vi "fft_demodulator.vi"(0 "Reset":bool, 5 "Config":T2={"IO params"={"Conversion"={"Rate"=4.0, "Num cards"=2, "Out channels"=4}, "Carriers"={"Phase shift"=180.0, "Levels"=[[0.8, 0.8, 0.8], [0.03, 0.03, 0.03]], "Delay samples"=73.15}, "TCP"={"Host"="192.168.1.15", "Port"=6666, "Buffering"=6, "Timeout"=6}, "Input channel sign"=[1, 1, 1]}, "High rate STFT"={"Win param"=101.5, "Window type"=61, "Win order"=2, "DFT size"=64, "Channels"=[7], "Oversample"=64}, "Low rate STFT"={"Win param"=120.0, "Window type"=61, "Win order"=8, "DFT size"=64, "Channels"=[7], "Oversample"=64}, "Filtering "=[]} {"Filtering"."Distortion"."Limit" format="%#_3p"; "Filtering"."Distortion"."LF cut" format="%#_3p"; "Filtering"."Kalman"."Measure noise" format="%#_3p"; "Filtering"."Kalman"."Process noise" format="%#_3p"; "Filtering"."Hum"."Limit" format="%#_3p"; "Filtering"."Hum"."Frequency" format="%#_4p"; "Low rate STFT"."Oversample" min=1 step=1; "Low rate STFT"."Channels" min=0 step=1; "Low rate STFT"."DFT size" min=1 step=1; "Low rate STFT"."Window type" items=["Rectangle"=0, "Hanning"=1, "Hamming"=2, "Blackman-Harris"=3, "Exact Blackman"=4, "Blackman"=5, "Flat Top"=6, "4 Term B-Harris "=7, "7 Term B-Harris"=8, "Low Sidelobe"=9, "Blackman Nuttall"=11, "Triangle"=30, "Bartlett-Hanning"=31, "Bohman"=32, "Parzen"=33, "Welch"=34, "Kaiser"=60, "Dolph-Chebyshev"=61, "Gaussian"=62]; "High rate STFT"."Oversample" min=1 step=1; "High rate STFT"."Channels" min=0 step=1; "High rate STFT"."DFT size" min=1 step=1; "High rate STFT"."Window type" items=["Rectangle"=0, "Hanning"=1, "Hamming"=2, "Blackman-Harris"=3, "Exact Blackman"=4, "Blackman"=5, "Flat Top"=6, "4 Term B-Harris "=7, "7 Term B-Harris"=8, "Low Sidelobe"=9, "Blackman Nuttall"=11, "Triangle"=30, "Bartlett-Hanning"=31, "Bohman"=32, "Parzen"=33, "Welch"=34, "Kaiser"=60, "Dolph-Chebyshev"=61, "Gaussian"=62]; "IO params"."Input channel sign" min=-1 max=1 step=1; "IO params"."Carriers"."Levels" min=0.0 step=0.1; "IO params"."Conversion"."Rate" format="%#_8g"}, 7 "Modulation info":T8={"Fs full"=0.0, "Fs high"=0.0, "Fs low"=0.0, "Read size"=0, "FFT size low"=5000, "df low"=5000.0, "High carriers"=[], "Low carriers"=[], "Hi channels at low"=[7]} {"Hi channels at low" min=0 step=1; "Low carriers" format="%#_6p"; "High carriers" format="%#_6p"}, 9 "Low carrier amplitudes":cdb[](array[numeric]) format="%#_3p", 12 "Raw data":dbl[](array[numeric]), 13 "Current/sensor index":i32 min=0 max=1 step=1) -> (10 "High carrier amplitudes":cdb[][](array[numeric]) format="%_3p", 15 "Trace channel out":T1)   [LabVIEW 2026]
uses:
  modulation_info.ctl
  ilemt_config.ctl
  system/IO_params.ctl
  stft_params.ctl
  <vilib>/Analysis/4window.llb/windowTd.ctl
  filter_params.ctl
  detrend_mode.ctl
  gui/trace_channel.ctl
  <vilib>/Analysis/NI_AALPro.lvlib
panel:
  out "DIstortion filter attenuation":dbl
  out "Distortion filter RMS":dbl[](array[numeric])
  out "Distortion filter":dbl[][](graph)
  # "This VI deals with high-rate demodulation and filtering for a single sensor axis."
  # "Rows are time (high carrier samples), columns are high rate source XYZ axis amplitudes."
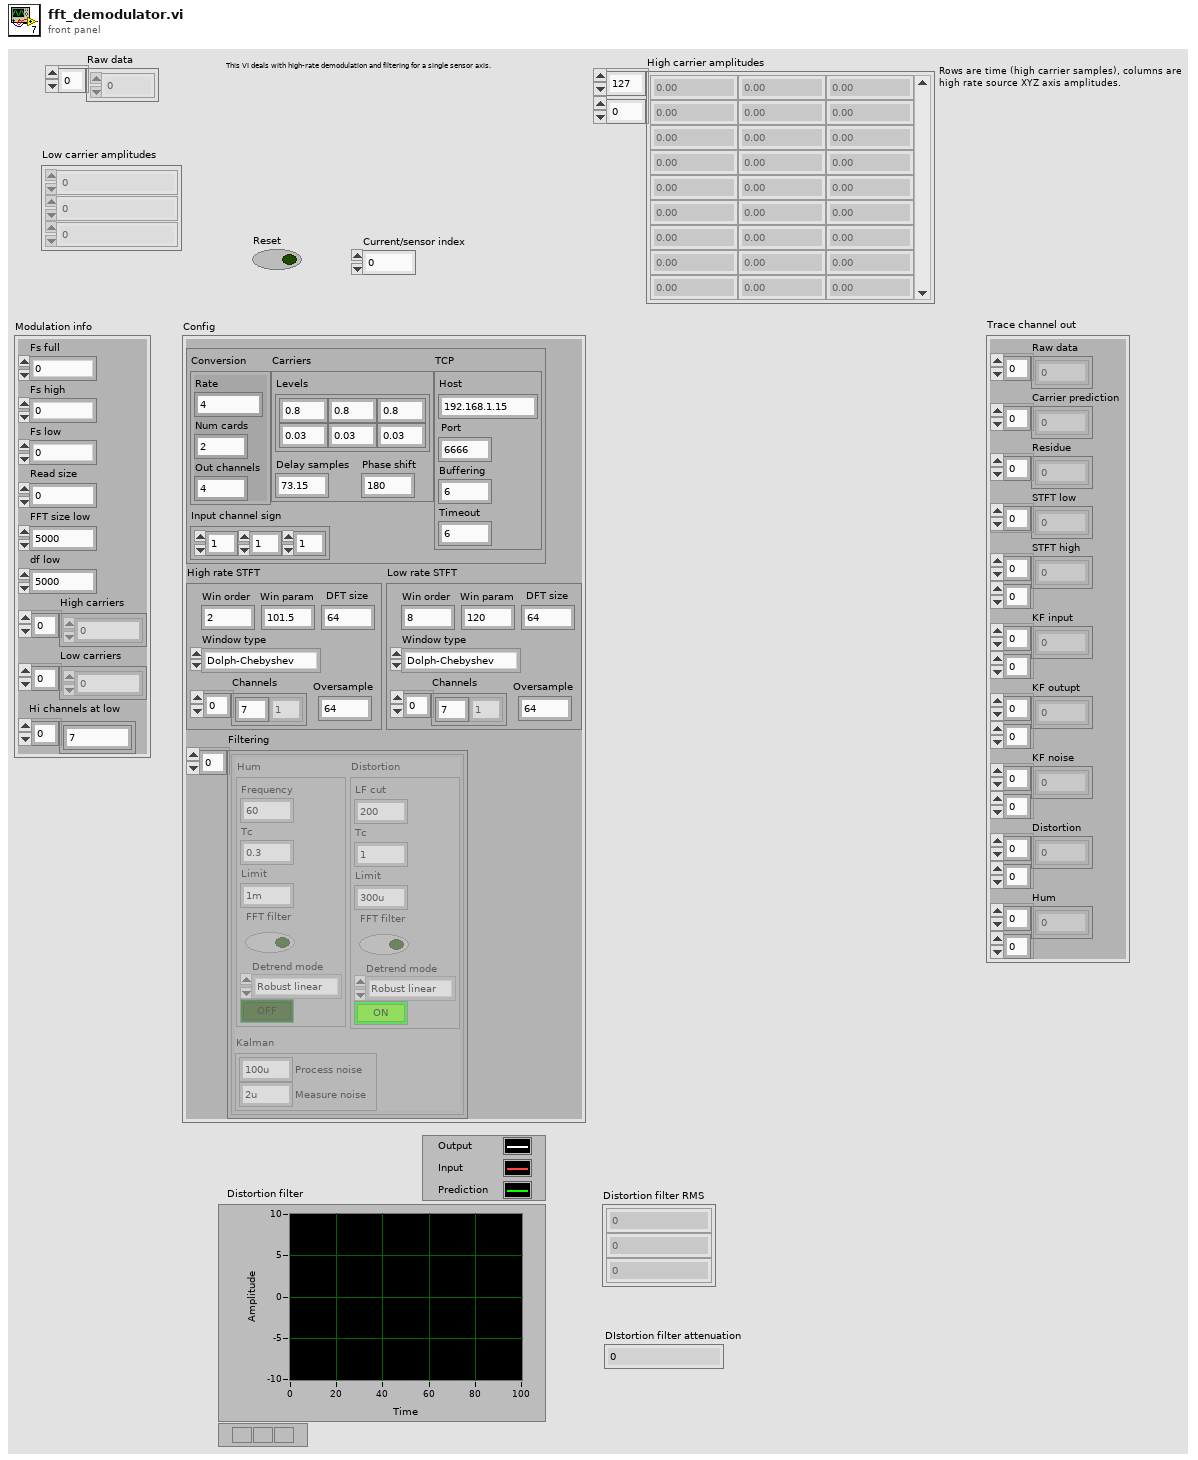
[diagram p1: front panel]
types:
  T1 = typedef "trace_channel.ctl" = cluster{"Raw data":dbl[], "Carrier prediction":dbl[], "Residue":dbl[], "STFT low":cdb[], "STFT high":cdb[][], "KF input":cdb[][], "KF outupt":cdb[][], "KF noise":dbl[][], "Distortion":cdb[][], "Hum":cdb[][]}
  T2 = typedef "ilemt_config.ctl" = cluster{"IO params":T3, "High rate STFT":T4, "Low rate STFT":T4, "Filtering ":T6[]}
  T3 = typedef "IO_params.ctl" = cluster{"Conversion":cluster{"Rate":dbl, "Num cards":u32, "Out channels":u32}, "Carriers":cluster{"Phase shift":dbl, "Levels":dbl[][], "Delay samples":dbl}, "TCP":cluster{"Host":string, "Port":i32, "Buffering":u32, "Timeout":u32}, "Input channel sign":i32[]}
  T4 = typedef "stft_params.ctl" = cluster{"Win param":dbl, "Window type":T5, "Win order":i32, "DFT size":i32, "Channels":i32[], "Oversample":i32}
  T5 = typedef "NI_AALPro.lvlib/windowTd.ctl" = u32
  T6 = typedef "filter_params.ctl" = cluster{"Hum":cluster{"Frequency":dbl, "Tc":dbl, "Limit":dbl, "FFT filter":bool, "Detrend mode":T7, "Enable":bool}, "Kalman":cluster{"Process noise":dbl, "Measure noise":dbl}, "Distortion":cluster{"LF cut":dbl, "Tc":dbl, "Limit":dbl, "FFT filter":bool, "Detrend mode":T7, "Enable":bool}}
  T7 = typedef "detrend_mode.ctl" = enum16{"Zero mean", "Linear", "Robust linear"}
  T8 = typedef "modulation_info.ctl" = cluster{"Fs full":dbl, "Fs high":dbl, "Fs low":dbl, "Read size":i32, "FFT size low":i32, "df low":dbl, "High carriers":dbl[], "Low carriers":dbl[], "Hi channels at low":i32[]}
  T9 = typedef "averaging_filter_params.ctl" = cluster{"Order":i32, "Time constant":dbl, "Detrend mode":T7, "TD amplitude limit":dbl, "FFT filter":bool, "Notch channels":i32[], "LF cutoff":i32, "FD amplitude limit":dbl}
  T10 = typedef "kalman_filter.ctl" = cluster{"A":T11, "B":T11, "H":T11, "Q":T11, "R":T11, "x":T11, "P":T11, "x lim":dbl[], "y lim":dbl[], "K":T11, "Converge count":i32}
  T11 = typedef "NI_Matrix.lvlib/RealMatrix.ctl" = dbl[][]
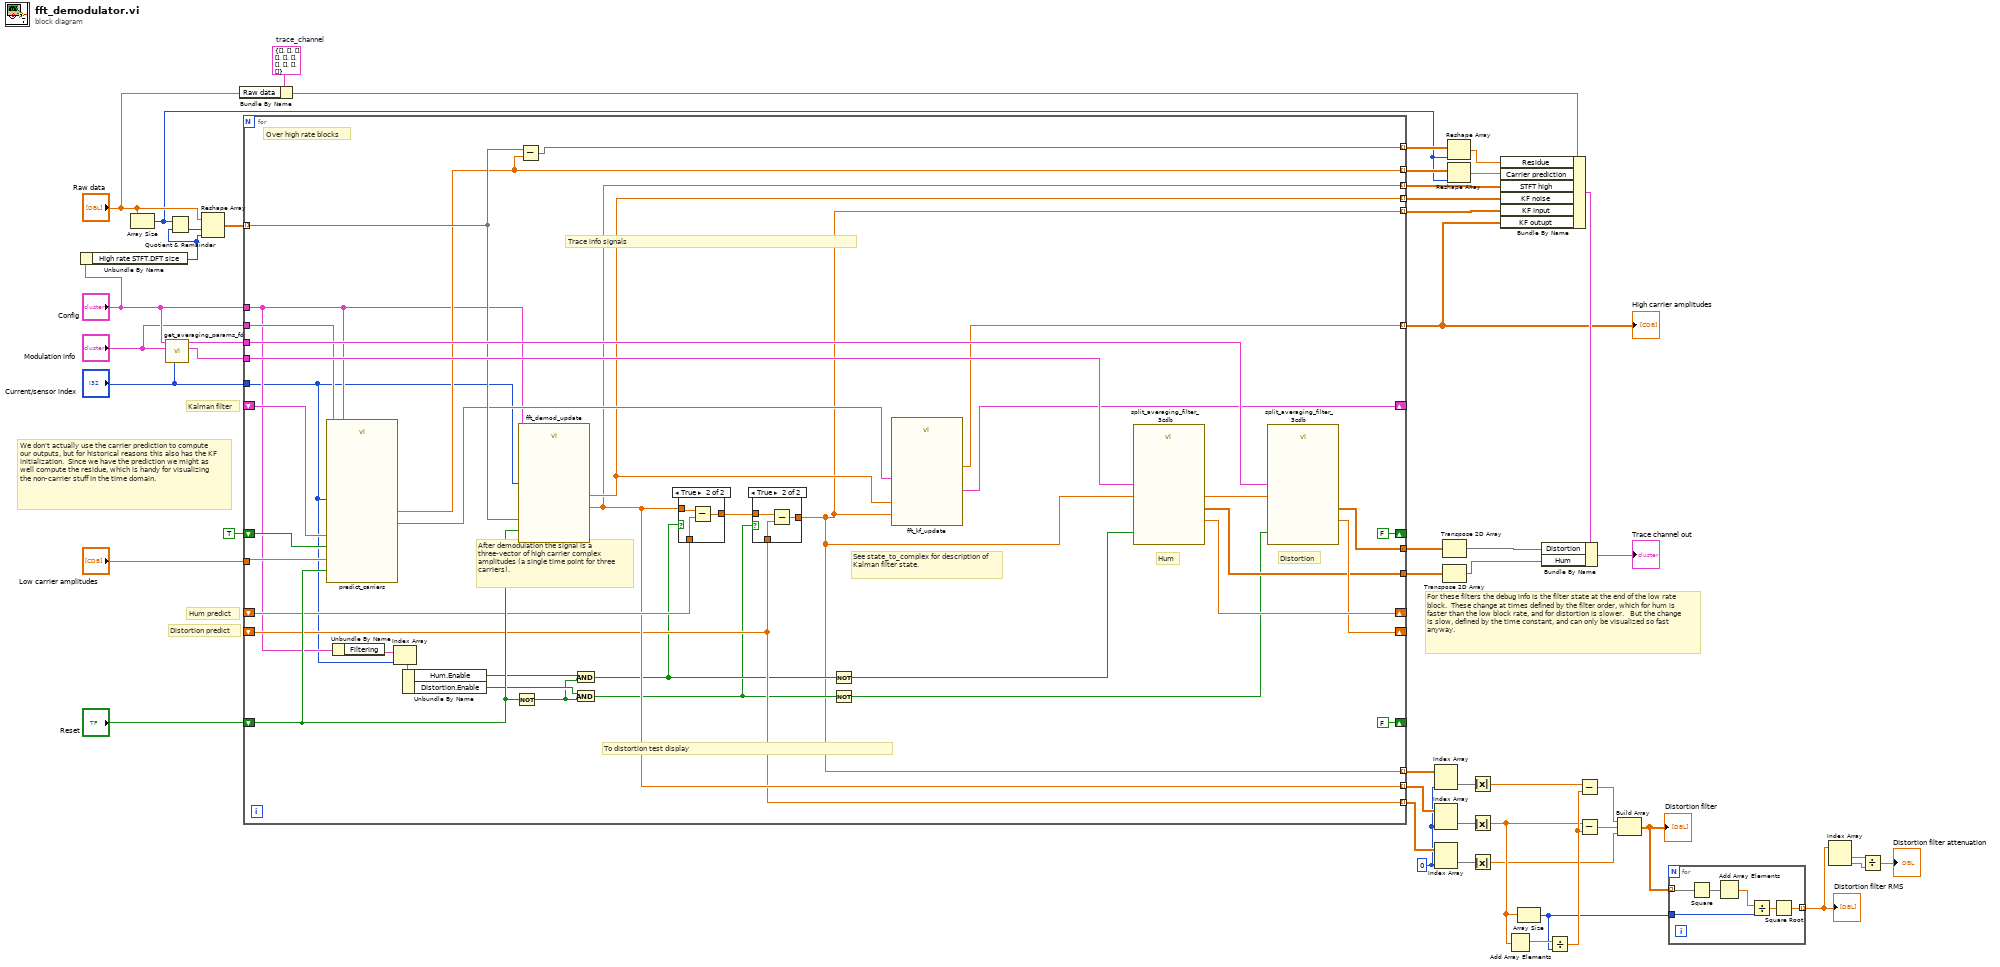
[diagram p0: block diagram]
diagram:
  w20 = 0 ("disabled index (col)")
  w39 = T1 {"Raw data"=[], "Carrier prediction"=[], "Residue"=[], "STFT low"=[], "STFT high"=[], "KF input"=[], "KF outupt"=[], "KF noise"=[], "Distortion"=[], "Hum"=[]}  # trace_channel
  # "Kalman filter"
  # "We don't actually use the carrier prediction to compute our outputs, but for historical reasons this also has the KF initialization.  Since we have the prediction we might as well compute the residue, which is handy for visualizing the non-carrier stuff in the time domain."
  # "For these filters the debug info is the filter state at the end of the low rate block.  These change at times defined by the filter order, which for hum is faster than the low block rate, and for distortion is slower.   But the change is slow, defined by the time constant, and can only be visualized so fast anyway."
  # "Distortion predict"
  # "Hum predict"
  n1 = Unbundle By Name("Config") -> ("High rate STFT.DFT size"=w42:i32)
  n2 = Array Size(array="Raw data") -> (size(s)=w29:i32)
  n3 = call "get_averaging_params_fd.vi"("Current/sensor index"="Current/sensor index", "Modulation info"="Modulation info", "Config"="Config") -> ("Hum params"=w47:T9, "Distortion params"=w49:T9)  [unwired: 7 in]
  n4 = Quotient & Remainder(x=w29, y=w42) -> (floor(x/y)=w45:i32)  [unwired: 1 out]
  n5 = Reshape Array("Raw data", w45, w42) -> (w46:dbl[][])
  n6 = Bundle By Name(cluster=w39, "Raw data"="Raw data") -> (w38:T1)
  n7 = for {
    tunnel: w49 -> [w83]
    tunnel: w46 -> [w71] mode=indexing
    tunnel: w47 -> [w82]
    shift-right: [FALSE ("Reset")] -> _
    shift-left: "Reset" -> [w85]
    shift-right: [w68] -> _
    shift-left: _ -> [w75]
    tunnel: "Config" -> [w53]
    tunnel: [w65] -> w35 mode=indexing
    shift-right: [w81] -> _
    shift-left: _ -> [w79]
    shift-right: [w80] -> _
    shift-left: _ -> [w62]
    tunnel: "Modulation info" -> [w76]
    tunnel: [w78] -> w4
    tunnel: [w77] -> w2
    tunnel: [w54] -> w36 mode=indexing
    shift-right: [FALSE ("Reset")] -> _
    shift-left: TRUE ("Reset") -> [w74]
    tunnel: "Low carrier amplitudes" -> [w72]
    tunnel: [w70] -> w32 mode=indexing
    tunnel: [w66] -> w30 mode=indexing
    tunnel: [w64] -> w27 mode=indexing
    tunnel: [w67] -> w26 mode=indexing
    tunnel: [w62] -> w23 mode=indexing
    tunnel: [w64] -> w22 mode=indexing
    tunnel: [w54] -> w21 mode=indexing
    tunnel: "Current/sensor index" -> [w50]
    # "Trace info signals"
    # "To distortion test display"
    # "After demodulation the signal is a three-vector of high carrier complex amplitudes (a single time point for three carriers)."
    # "See state_to_complex for description of Kalman filter state."
    # "Over high rate blocks"
    # "Distortion"
    # "Hum"
    n8 = call "predict_carriers.vi"("Current/sensor index"=w50, "Modulation info"=w76, "Low rate block start"=w74, "Low carrier amplitudes"=w72, "KF in"=w75, "Reset"=w85, "Config"=w53) -> ("KF out"=w69:T10, "Predicted carriers"=w66:dbl[])  [unwired: 3 in]
    n9 = Unbundle By Name(w53) -> ("Filtering"=w52:T6[])
    n10 = Index Array(array=w52, index=w50) -> (element=w51:T6)
    n11 = Unbundle By Name(w51) -> ("Hum.Enable"=w61:bool, "Distortion.Enable"=w60:bool)
    n12 = Not(x=w85) -> (.not. x?=w59:bool)
    n13 = call "fft_demod_update.vi"("Current/sensor index"=w50, "Reset"=w85, "Config"=w53, "Signal"=w71) -> ("Measure noise RMS"=w67:dbl[], "Measurement amplitudes"=w64:cdb[])  [unwired: 6 in]
    n14 = Subtract(x=w71, y=w66) -> (x-y=w70:dbl[])
    n15 = And(x=w61, y=w59) -> (x .and. y?=w58:bool)
    n16 = And(x=w60, y=w59) -> (x .and. y?=w57:bool)
    n17 = case shown="True" w58 {
      tunnel: [w90 w93] -> w63
      tunnel: w79 -> [_ w92]
      tunnel: w64 -> [w90 w91]
      frame False {
      }
      frame True {
        n18 = Subtract(x=w91, y=w92) -> (x-y=w93:cdb[])
      }
    }
    n19 = case shown="True" w57 {
      tunnel: w63 -> [w86 w89]
      tunnel: w62 -> [_ w88]
      tunnel: [w86 w87] -> w54
      frame False {
      }
      frame True {
        n20 = Subtract(x=w89, y=w88) -> (x-y=w87:cdb[])
      }
    }
    n21 = Not(x=w58) -> (.not. x?=w55:bool)
    n22 = Not(x=w57) -> (.not. x?=w56:bool)
    n23 = call "fft_kf_update.vi"("Measurement"=w54, "Measure noise RMS"=w67, "KF in"=w69) -> ("KF out"=w68:T10, "KF estimate"=w65:cdb[])  [unwired: 7 in]
    n24 = call "split_averaging_filter_3cdb.vi"("Reset"=w55, "Parameters"=w82, "Error"=w54) -> ("Model"=w77:cdb[][], "Prediction"=w81:cdb[])  [unwired: 7 in]
    n25 = call "split_averaging_filter_3cdb.vi"("Reset"=w56, "Parameters"=w83, "Error"=w54) -> ("Model"=w78:cdb[][], "Prediction"=w80:cdb[])  [unwired: 7 in]
  }
  "High carrier amplitudes" <- w35
  n26 = Index Array(array=w21, index (col)=w20) -> (element=w15:cdb[])  [unwired: 1 in]
  n27 = Index Array(array=w22, index (col)=w20) -> (element=w14:cdb[])  [unwired: 1 in]
  n28 = Index Array(array=w23, index (col)=w20) -> (element=w12:cdb[])  [unwired: 1 in]
  n29 = Transpose 2D Array(2D array=w4) -> (transposed array=w3:cdb[][])
  n30 = Transpose 2D Array(2D array=w2) -> (transposed array=w1:cdb[][])
  n31 = Reshape Array(w32, w29) -> (w31:dbl[])
  n32 = Reshape Array(w30, w29) -> (w28:dbl[])
  n33 = Absolute Value(x=w15) -> (abs(x)=w10:dbl[])
  n34 = Absolute Value(x=w14) -> (abs(x)=w13:dbl[])
  n35 = Absolute Value(x=w12) -> (abs(x)=w11:dbl[])
  n36 = Bundle By Name(cluster=w38, "Residue"=w31, "Carrier prediction"=w28, "STFT high"=w27, "KF noise"=w26, "KF input"=w36, "KF outupt"=w35) -> (w41:T1)
  n37 = Add Array Elements(numeric array=w13) -> (sum=w25:dbl)
  n38 = Array Size(array=w13) -> (size(s)=w16:i32)
  n39 = Bundle By Name(cluster=w41, "Distortion"=w3, "Hum"=w1) -> (→"Trace channel out":T1)
  n40 = Divide(x=w25, y=w16) -> (x/y=w19:dbl)
  n41 = Subtract(x=w10, y=w19) -> (x-y=w18:dbl[])
  n42 = Subtract(x=w13, y=w19) -> (x-y=w24:dbl[])
  n43 = Build Array(w18, w24, w11) -> (w17:dbl[][])
  "Distortion filter" <- w17
  n44 = for {
    tunnel: w17 -> [w98] mode=indexing
    tunnel: w16 -> [w96]
    tunnel: [w94] -> w9 mode=indexing
    n45 = Square(x=w98) -> (x^2=w97:dbl[])
    n46 = Add Array Elements(numeric array=w97) -> (sum=w99:dbl)
    n47 = Divide(x=w99, y=w96) -> (x/y=w95:dbl)
    n48 = Square Root(x=w95) -> (sqrt(x)=w94:dbl)
  }
  "Distortion filter RMS" <- w9
  n49 = Index Array(array=w9) -> (element #1=w7:dbl, element #2=w6:dbl)  [unwired: 2 in]
  n50 = Divide(x=w7, y=w6) -> (x/y=→"DIstortion filter attenuation":dbl)
